vi "WPI_ADIS16448Open.vi"(0 "Controller":T3, 1 "SPI Clock Rate (Hz)":dbl=2000000.0, 9 "Sample Mode":T9, 11 "error in":errorcluster) -> (4 "ADIS16448DevRef":T1 {"Registers to Read" items=["XGYRO_OUT"=4, "YGYRO_OUT"=6, "ZGYRO_OUT"=8, "XACCL_OUT"=10, "YACCL_OUT"=12, "ZACCL_OUT"=14, "XMAGN_OUT"=16, "YMAGN_OUT"=18, "ZMAGN_OUT"=20, "BARO_OUT"=22, "TEMP_OUT"=24]}, 15 "error out":errorcluster)   [LabVIEW 2014, in "ADIS16448.lvlib"]
uses:
  ADIS16448.lvlib
  <vilib>/Rock Robotics/SystemInterfaces/Typedef/FPGA_TypedefDigitalModule.ctl
  Typedef/WPI_ADIS16448SampleMode.ctl
  Typedef/WPI_ADIS16448Ref.ctl
  <vilib>/Rock Robotics/WPI/SPI/WPI_SPIDevRef.ctl
  <vilib>/Rock Robotics/SystemInterfaces/spilib/spi_bus.ctl
  <vilib>/Rock Robotics/SystemInterfaces/CounterEncoderSourceConvertion/FPGA_CounterEncoderSourceConvertionLVSourceType.ctl
  <vilib>/Rock Robotics/SystemInterfaces/DIO/FPGA_DIODigitalSourceChannel.ctl
  <vilib>/Rock Robotics/SystemInterfaces/AnalogTrigger/FPGA_AnalogTriggerIndex.ctl
  <vilib>/Rock Robotics/SystemInterfaces/AnalogTrigger/FPGA_AnalogTriggerOutType.ctl
  Typedef/WPI_ADIS16448DataRegisters.ctl
  Typedef/WPI_ADIS16448ReadingsDVR.ctl
  Typedef/WPI_ADIS16448Readings.ctl
  <vilib>/Rock Robotics/SystemInterfaces/Interrupt/FPGA_InterruptRef.ctl
  <vilib>/Rock Robotics/SystemInterfaces/Interrupt/FPGA_InterruptIndex.ctl
  <vilib>/Rock Robotics/SystemInterfaces/DIO/FPGA_DIOChannel.ctl
  <vilib>/Rock Robotics/WPI/Counter/WPI_CounterDigitalInputToDigitalSource.vi
  <vilib>/Rock Robotics/SystemInterfaces/CounterEncoderSourceConvertion/FPGA_CounterEncoderSourceConvertionLVSourceTypeToFPGAType.vi
  <vilib>/Rock Robotics/WPI/Interrupt/WPI_InterruptCache.vi
  <vilib>/Rock Robotics/SystemInterfaces/Interrupt/FPGA_InterruptWriteConfiguration.vi
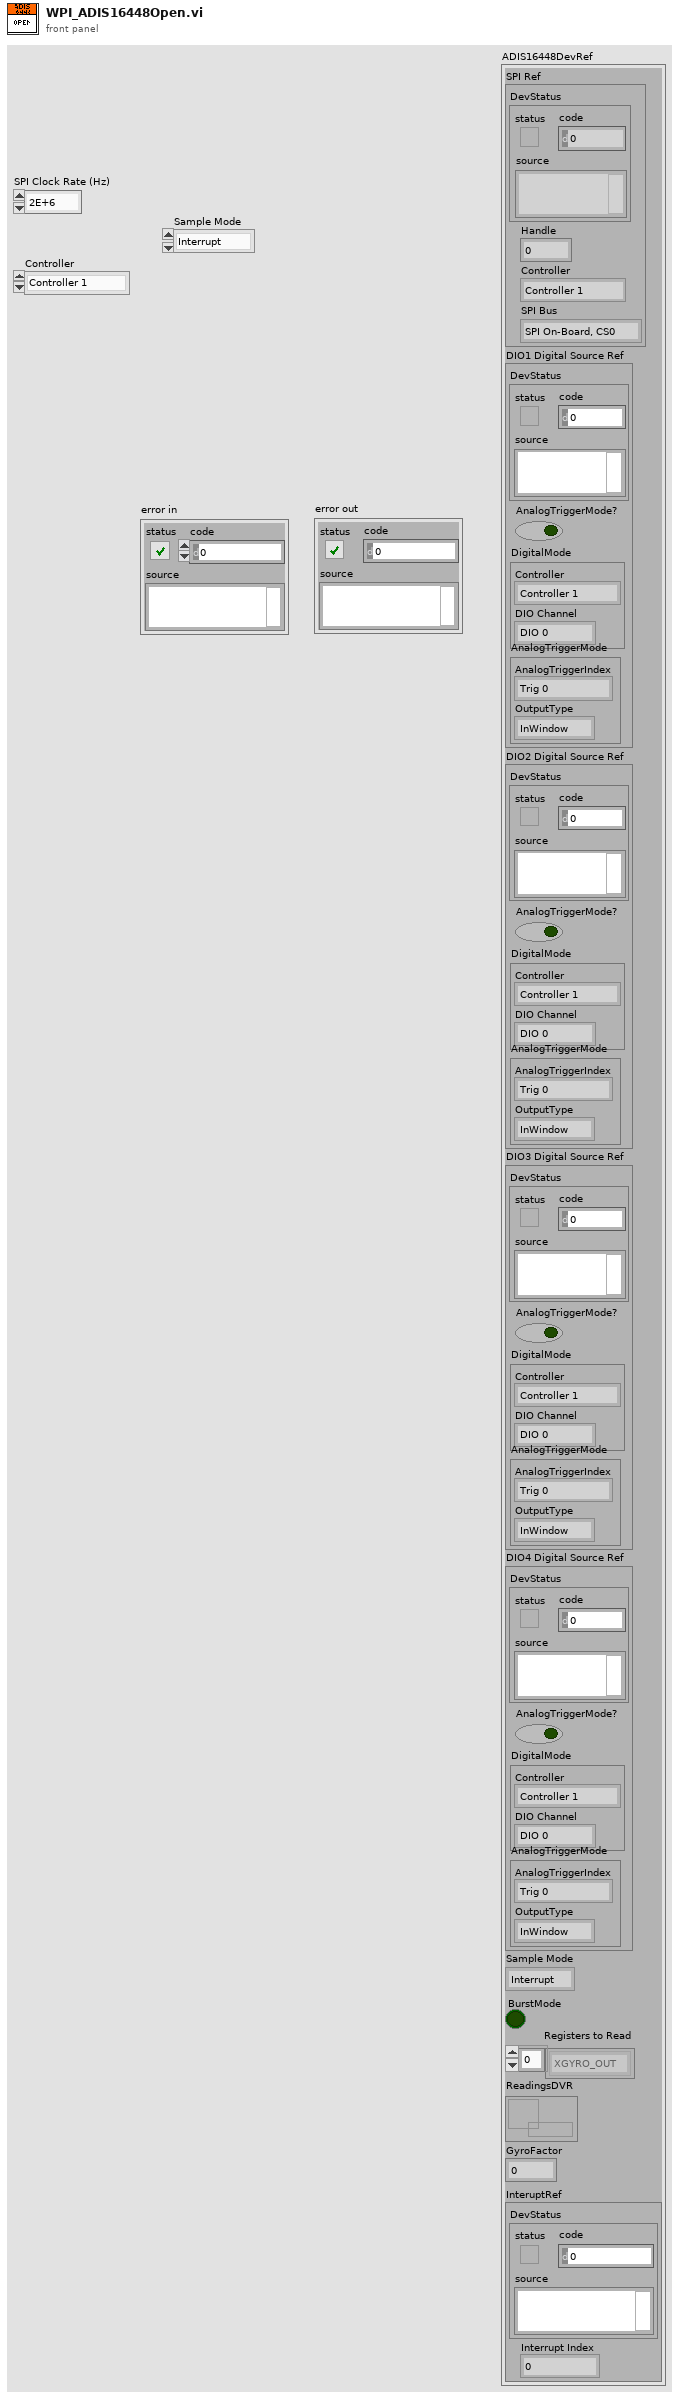
[diagram p1: front panel]
types:
  T1 = typedef "ADIS16448.lvlib/WPI_ADIS16448Ref.ctl" = cluster{"SPI Ref":T2, "DIO1 Digital Source Ref":T5, "DIO2 Digital Source Ref":T5, "DIO3 Digital Source Ref":T5, "DIO4 Digital Source Ref":T5, "Sample Mode":T9, "BurstMode":bool, "Registers to Read":T10[], "ReadingsDVR":T11, "GyroFactor":dbl, "InteruptRef":T12}
  T2 = typedef "WPI_SPIDevRef.ctl" = cluster{"DevStatus":errorcluster, "Handle":i32, "Controller":T3, "SPI Bus":T4}
  T3 = typedef "FPGA_TypedefDigitalModule.ctl" = enum16{"Controller 1"}
  T4 = typedef "spi_bus.ctl" = enum16{"SPI On-Board, CS0", "SPI On-Board, CS1", "SPI On-Board, CS2", "SPI On-Board, CS3", "SPI MXP", "Invalid"}
  T5 = typedef "FPGA_CounterEncoderSourceConvertionLVSourceType.ctl" = cluster{"DevStatus":errorcluster, "AnalogTriggerMode?":bool, "DigitalMode":cluster{"Controller":T3, "DIO Channel":T6}, "AnalogTriggerMode":cluster{"AnalogTriggerIndex":T7, "OutputType":T8}}
  T6 = typedef "FPGA_DIODigitalSourceChannel.ctl" = enum8{"DIO 0", "DIO 1", "DIO 2", "DIO 3", "DIO 4", "DIO 5", "DIO 6", "DIO 7", "DIO 8", "DIO 9", "DIO MXP 0", "DIO MXP 1", "DIO MXP 2", "DIO MXP 3", "DIO MXP 4", "DIO MXP 5", "DIO MXP 6", "DIO MXP 7", "DIO MXP 8", "DIO MXP 9", "DIO MXP 10", "DIO MXP 11", "DIO MXP 12", "DIO MXP 13", "DIO MXP 14", "DIO MXP 15", "Disabled"}
  T7 = typedef "FPGA_AnalogTriggerIndex.ctl" = enum8{"Trig 0", "Trig 1", "Trig 2", "Trig 3", "Trig 4", "Trig 5", "Trig 6", "Trig 7", "Invalid"}
  T8 = typedef "FPGA_AnalogTriggerOutType.ctl" = enum16{"InWindow", "TriggerState", "Rising", "Falling"}
  T9 = typedef "ADIS16448.lvlib/WPI_ADIS16448SampleMode.ctl" = enum16{"Interrupt", "Polled"}
  T10 = typedef "ADIS16448.lvlib/WPI_ADIS16448DataRegisters.ctl" = u16
  T11 = typedef "ADIS16448.lvlib/WPI_ADIS16448ReadingsDVR.ctl" = refnum<data-value>
  T12 = typedef "FPGA_InterruptRef.ctl" = cluster{"DevStatus":errorcluster, "Interrupt Index":T13}
  T13 = typedef "FPGA_InterruptIndex.ctl" = enum8{"0", "1", "2", "3", "4", "5", "6", "7", "Invalid"}
  T14 = typedef "FPGA_DIOChannel.ctl" = enum8{"DIO 0", "DIO 1", "DIO 2", "DIO 3", "DIO 4", "DIO 5", "DIO 6", "DIO 7", "DIO 8", "DIO 9", "DIO MXP 0", "DIO MXP 1", "DIO MXP 2", "DIO MXP 3", "DIO MXP 4", "DIO MXP 5", "DIO MXP 6", "DIO MXP 7", "DIO MXP 8", "DIO MXP 9", "DIO MXP 10", "DIO MXP 11", "DIO MXP 12", "DIO MXP 13", "DIO MXP 14", "DIO MXP 15", "Invalid"}
  T15 = cluster{"DIO2 Channel":T14, "DIO3 Channel":T14, "DIO4 Channel":T14}
  T16 = typedef "WPI_DigitalInputDevRef.ctl" = cluster{"DevStatus":errorcluster, "DIO Channel":T14, "Controller":T3}
  T17 = typedef "WPI_InterruptRef.ctl" = cluster{"DevStatus":errorcluster, "InterruptIndex":T13}
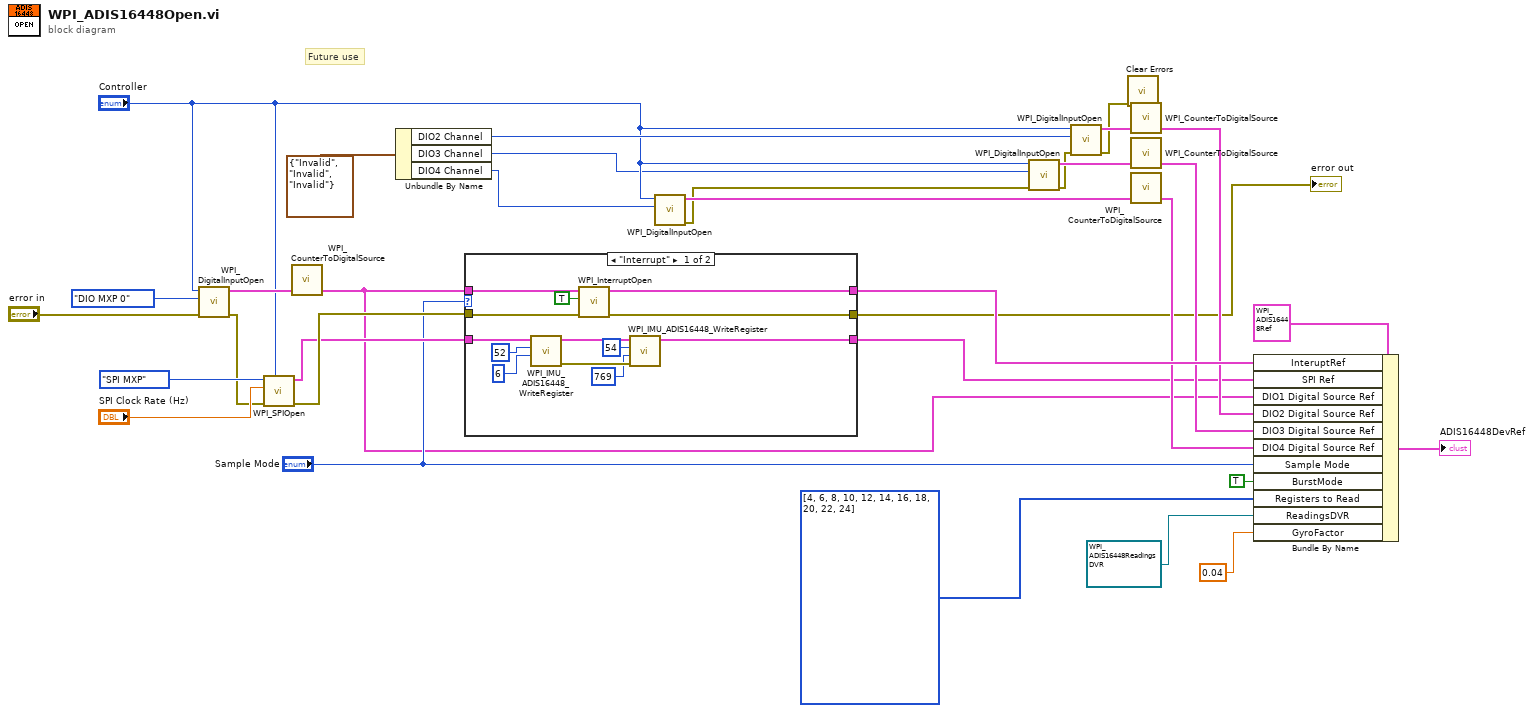
[diagram p0: block diagram]
diagram:
  w8 = T10[] [4, 6, 8, 10, 12, 14, 16, 18, 20, 22, 24] items=["XGYRO_OUT"=4, "YGYRO_OUT"=6, "ZGYRO_OUT"=8, "XACCL_OUT"=10, "YACCL_OUT"=12, "ZACCL_OUT"=14, "XMAGN_OUT"=16, "YMAGN_OUT"=18, "ZMAGN_OUT"=20, "BARO_OUT"=22, "TEMP_OUT"=24] ("Registers to Read")
  # "Future use"
  n1 = call <vilib>:"WPI_DigitalInputOpen.vi"("error in (no error)"="error in", "DIO Channel"=FPGA_DIOChannel."DIO MXP 0" ("DIO1 Channel"), "Controller"="Controller") -> ("error out"=w16:errorcluster, "DigitalInputDevRef"=w30:T16)  [unwired: 7 in]
  n2 = call <vilib>:"WPI_SPIOpen.vi"("Controller"="Controller", "error in"=w16, "Clock Rate (Hz)"="SPI Clock Rate (Hz)", "SPI Bus"=spi_bus."SPI MXP" ("SPI Port")) -> ("error out"=w15:errorcluster, "SPIDevRef"=w5:T2)  [unwired: 6 in]
  n3 = call-poly <vilib>:"WPI_CounterToDigitalSource.vi"("DigitalInputDevRef"=w30) -> ("Digital Source"=w1:T5)  [unwired: 6 in]
  n4 = Unbundle By Name(T15 {"DIO2 Channel"=enum."Invalid", "DIO3 Channel"=enum."Invalid", "DIO4 Channel"=enum."Invalid"} ("Extra Channels")) -> ("DIO2 Channel"=w27:T14, "DIO3 Channel"=w25:T14, "DIO4 Channel"=w24:T14)
  n5 = case shown="\"Interrupt\"" "Sample Mode" {
    tunnel: [w46 _] -> w31
    tunnel: w1 -> [w45 _]
    tunnel: w15 -> [w44 w48]
    tunnel: [w43 w48] -> w7
    tunnel: w5 -> [w41 w47]
    tunnel: [w34 w47] -> w4
    frame "Interrupt" {
      n6 = call "WPI_IMU_ADIS16448_WriteRegister.vi"("Data"=u16 6, "Address"=u16 52, "SPIDevRef in"=w41) -> ("error out"=w38:errorcluster, "SPIDevRef out"=w37:T2)  [unwired: 7 in]
      n7 = call <vilib>:"WPI_InterruptOpen.vi"("error in (no error)"=w44, "Rising Edge"=TRUE, "Source"=w45) -> ("error out"=w43:errorcluster, "InterruptRef"=w46:T17)  [unwired: 7 in]
      n8 = call "WPI_IMU_ADIS16448_WriteRegister.vi"("error in"=w38, "Data"=u16 769, "Address"=u16 54, "SPIDevRef in"=w37) -> ("SPIDevRef out"=w34:T2)  [unwired: 6 in, 1 out]
    }
    frame "Polled", Default {
    }
  }
  "error out" <- w7
  n9 = call <vilib>:"WPI_DigitalInputOpen.vi"("DIO Channel"=w24, "Controller"="Controller") -> ("error out"=w14:errorcluster, "DigitalInputDevRef"=w20:T16)  [unwired: 8 in]
  n10 = call <vilib>:"WPI_DigitalInputOpen.vi"("error in (no error)"=w14, "DIO Channel"=w25, "Controller"="Controller") -> ("error out"=w13:errorcluster, "DigitalInputDevRef"=w21:T16)  [unwired: 7 in]
  n11 = call <vilib>:"WPI_DigitalInputOpen.vi"("error in (no error)"=w13, "DIO Channel"=w27, "Controller"="Controller") -> ("error out"=w6:errorcluster, "DigitalInputDevRef"=w23:T16)  [unwired: 7 in]
  n12 = call <vilib>:"Clear Errors.vi"("error in (no error)"=w6) -> ()  [unwired: 5 in, 2 out]
  n13 = call-poly <vilib>:"WPI_CounterToDigitalSource.vi"("DigitalInputDevRef"=w23) -> ("Digital Source"=w22:T5)  [unwired: 6 in]
  n14 = call-poly <vilib>:"WPI_CounterToDigitalSource.vi"("DigitalInputDevRef"=w21) -> ("Digital Source"=w19:T5)  [unwired: 6 in]
  n15 = call-poly <vilib>:"WPI_CounterToDigitalSource.vi"("DigitalInputDevRef"=w20) -> ("Digital Source"=w18:T5)  [unwired: 6 in]
  n16 = Bundle By Name(cluster=T1 {"SPI Ref"={"DevStatus"={"status"=FALSE, "code"=0, "source"=""}, "Handle"=0, "Controller"=enum."Controller 1", "SPI Bus"=enum."SPI On-Board, CS0"}, "DIO1 Digital Source Ref"={"DevStatus"={"status"=FALSE, "code"=0, "source"=""}, "AnalogTriggerMode?"=FALSE, "DigitalMode"={"Controller"=enum."Controller 1", "DIO Channel"=enum."DIO 0"}, "AnalogTriggerMode"={"AnalogTriggerIndex"=enum."Trig 0", "OutputType"=enum."InWindow"}}, "DIO2 Digital Source Ref"={"DevStatus"={"status"=FALSE, "code"=0, "source"=""}, "AnalogTriggerMode?"=FALSE, "DigitalMode"={"Controller"=enum."Controller 1", "DIO Channel"=enum."DIO 0"}, "AnalogTriggerMode"={"AnalogTriggerIndex"=enum."Trig 0", "OutputType"=enum."InWindow"}}, "DIO3 Digital Source Ref"={"DevStatus"={"status"=FALSE, "code"=0, "source"=""}, "AnalogTriggerMode?"=FALSE, "DigitalMode"={"Controller"=enum."Controller 1", "DIO Channel"=enum."DIO 0"}, "AnalogTriggerMode"={"AnalogTriggerIndex"=enum."Trig 0", "OutputType"=enum."InWindow"}}, "DIO4 Digital Source Ref"={"DevStatus"={"status"=FALSE, "code"=0, "source"=""}, "AnalogTriggerMode?"=FALSE, "DigitalMode"={"Controller"=enum."Controller 1", "DIO Channel"=enum."DIO 0"}, "AnalogTriggerMode"={"AnalogTriggerIndex"=enum."Trig 0", "OutputType"=enum."InWindow"}}, "Sample Mode"=enum."Interrupt", "BurstMode"=FALSE, "Registers to Read"=[], "ReadingsDVR"=refnum, "GyroFactor"=0.0, "InteruptRef"={"DevStatus"={"status"=FALSE, "code"=0, "source"=""}, "Interrupt Index"=enum."0"}}, "InteruptRef"=w31, "SPI Ref"=w4, "DIO1 Digital Source Ref"=w1, "DIO2 Digital Source Ref"=w22, "DIO3 Digital Source Ref"=w19, "DIO4 Digital Source Ref"=w18, "Sample Mode"="Sample Mode", "BurstMode"=TRUE, "Registers to Read"=w8, "ReadingsDVR"=T11 refnum, "GyroFactor"=0.04) -> (→"ADIS16448DevRef":T1)
